vi "Main On Load Action VI.vi"(8 "error in (no error)":errorcluster, 11 "Device Item Ref in":T1 format="%.0x") -> (0 "error out":errorcluster, 3 "Device Item Ref out":T1 format="%.0x")   [LabVIEW 2014, in "AIT 1553 Custom Device.lvlib"]
uses:
  AIT 1553 Custom Device.lvlib
  <vilib>/NI Veristand/Custom Device API/Custom Device Item Ref.ctl
  <vilib>/NI Veristand/Custom Device API/Custom Device Path Data.ctl
  <vilib>/NI Veristand/Custom Device API/Custom Device Supported Target.ctl
  <vilib>/NI Veristand/Custom Device API/Path Specification.ctl
  <vilib>/NI Veristand/Custom Device API/Path Type.ctl
  <vilib>/NI Veristand/Custom Device API/Custom Device Execution Mode.ctl
  <vilib>/NI Veristand/Custom Device API/Custom Device API.lvlib
  Controls and Global/Global.vi
  NationalInstruments.VeriStand.SystemDefinitionAPI
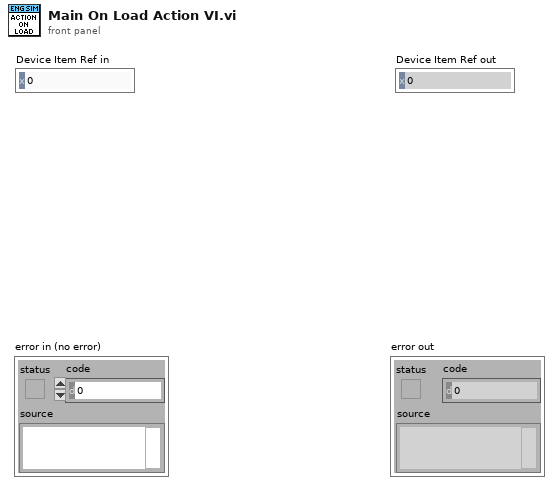
[diagram p1: front panel]
types:
  T1 = typedef "Custom Device API.lvlib/Custom Device Item Ref.ctl" = u64
  T2 = typedef "Custom Device API.lvlib/Path Specification.ctl" = cluster{"Path":path, "Type":T3}
  T3 = typedef "Custom Device API.lvlib/Path Type.ctl" = enum16{"Absolute", "To Base", "To Common Data Dir", "To Application Data Dir"}
  T4 = typedef "Custom Device API.lvlib/Custom Device Execution Mode.ctl" = enum16{"Asynchronous", "Inline HW Interface", "Inline Model Interface", "Inline Timing and Sync", "Asynchronous Timing and Sync"}
  T5 = typedef "Custom Device API.lvlib/Custom Device Supported Target.ctl" = enum16{"All", "PharLap", "VxWorks", "Windows", "PharLap & Windows", "PharLap & VxWorks", "VxWorks & Windows"}
  T6 = typedef "Custom Device API.lvlib/Custom Device Path Data.ctl" = cluster{"SupportedTarget":T5, "Source":T2, "RT Destination":path}
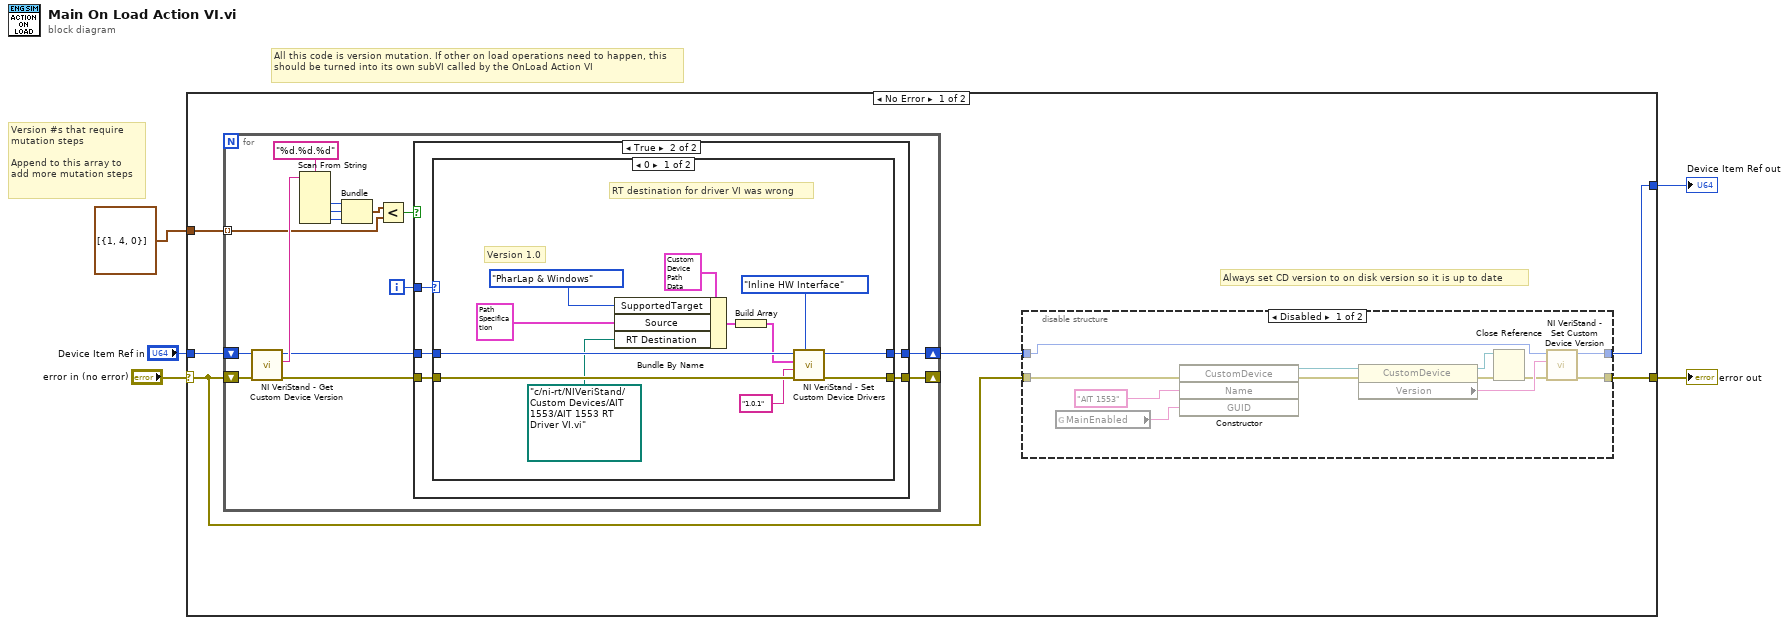
[diagram p0: block diagram]
diagram:
  # "All this code is version mutation. If other on load operations need to happen, this should be turned into its own subVI called by the OnLoad Action VI"
  # "Version #s that require\nmutation steps\n\nAppend to this array to\nadd more mutation steps"
  n1 = case shown="No Error" "error in (no error)" {
    selector: "error in (no error)" -> [w6 w63]
    tunnel: [w8 w63] -> w4
    tunnel: "Device Item Ref in" -> [w10 w62]
    tunnel: [w7 w62] -> w2
    tunnel: cluster{i32, i32, i32}[] [{1, 4, 0}] -> [w11 _]
    frame No Error {
      # "Always set CD version to on disk version so it is up to date"
      n2 = for {
        tunnel: w11 -> [w27] mode=indexing
        shift-right: [w31] -> _
        shift-left: w6 -> [w36]
        shift-right: [w29] -> w9
        shift-left: w10 -> [w35]
        i -> [w28]
        n3 = call <vilib>:"NI VeriStand - Get Custom Device Version.vi"("error in (no error)"=w36, "Device Ref in"=w35) -> ("error out"=w32:errorcluster, "Value"=w34:string, "Device Ref out"=w30:T1)  [unwired: 7 in]
        n4 = Scan From String(format string="%d.%d.%d", input string=w34) -> (output 1=w38:i32, output 2=w39:i32, output 3=w26:i32)  [unwired: 5 in, 3 out]
        n5 = Bundle(w38, w39, w26) -> (w40:cluster{i32, i32, i32})  [unwired: 1 in]
        n6 = Less?(x=w40, y=w27) -> (x < y?=w33:bool)
        n7 = case shown="True" w33 {
          tunnel: w32 -> [w42 w47]
          tunnel: [w42 w46] -> w31
          tunnel: w30 -> [w41 w43]
          tunnel: [w41 w44] -> w29
          tunnel: w28 -> [_ w45]
          frame False {
          }
          frame True {
            n8 = case shown="0" w45 {
              tunnel: w47 -> [w57 w61]
              tunnel: [w50 w61] -> w46
              tunnel: [w59 w60] -> w44
              tunnel: w43 -> [w56 w60]
              frame 0 {
                # "RT destination for driver VI was wrong"
                # "Version 1.0"
                n9 = Bundle By Name(cluster=T6 {"SupportedTarget"=enum."All", "Source"={"Path"=path "", "Type"=enum."Absolute"}, "RT Destination"=path ""} ("Driver VI Path"), "SupportedTarget"=Custom_Device_Supported_Target."PharLap & Windows", "Source"=T2 {"Path"=path "Custom Devices/AIT 1553/AIT 1553 RT Driver VI.vi", "Type"=enum."To Common Data Dir"}, "RT Destination"=path "c:/ni-rt/NIVeriStand/Custom Devices/AIT 1553/AIT 1553 RT Driver VI.vi") -> (w54:T6)
                n10 = Build Array(w54) -> (w53:T6[])
                n11 = call <vilib>:"NI VeriStand - Set Custom Device Drivers.vi"("Execution mode"=Custom_Device_Execution_Mode."Inline HW Interface", "error in (no error)"=w57, "Version"="1.0.1" ("format string"), "Driver VI"=w53, "Device Ref in"=w56) -> ("error out"=w50:errorcluster, "Device Ref out"=w59:T1)  [unwired: 5 in]
              }
              frame Default {
              }
            }
          }
        }
      }
      n12 = disable-structure shown="Disabled" {
        disable-tunnel: w9 -> [w23 w24]
        disable-tunnel: w6 -> [w22 w25]
        disable-tunnel: [w14 w25] -> w8
        disable-tunnel: [w13 w24] -> w7
        frame Disabled {
          n13 = global read "Global.vi" "MainEnabled"() -> (w12:string)
          n14 = constructor class="CustomDevice"(error in=w22, "Name"="AIT 1553", "GUID"=w12) -> (reference out=w20:refnum<k24>, error out=w19:errorcluster)  [unwired: 2 in, 3 out]
          n15 = property class="CustomDevice"(reference=w20, error in=w19) -> (reference out=w17:refnum<k24>, error out=w18:errorcluster, "Version"=w16:string)
          n16 = Close Reference(reference=w17, error in (no error)=w18) -> (error out=w15:errorcluster)
          n17 = call <vilib>:"NI VeriStand - Set Custom Device Version.vi"("error in (no error)"=w15, "Value"=w16, "Device Ref in"=w23) -> ("error out"=w14:errorcluster, "Device Ref out"=w13:T1)  [unwired: 7 in]
        }
        frame Enabled {
        }
      }
    }
    frame Error {
    }
  }
  "error out" <- w4
  "Device Item Ref out" <- w2
